vi "InflationApparatus.vi"() -> ()   [LabVIEW 2020]
panel:
  in  "ctrl array":refnum<vi>[](array[refnum])
  in  "camera calibration switch":bool
  in  "force calibration switch":bool
  in  "inflation test switch":bool=TRUE
  in  "dynamic controls":T1(tab)
  in  "stop":bool
  out "current state":string
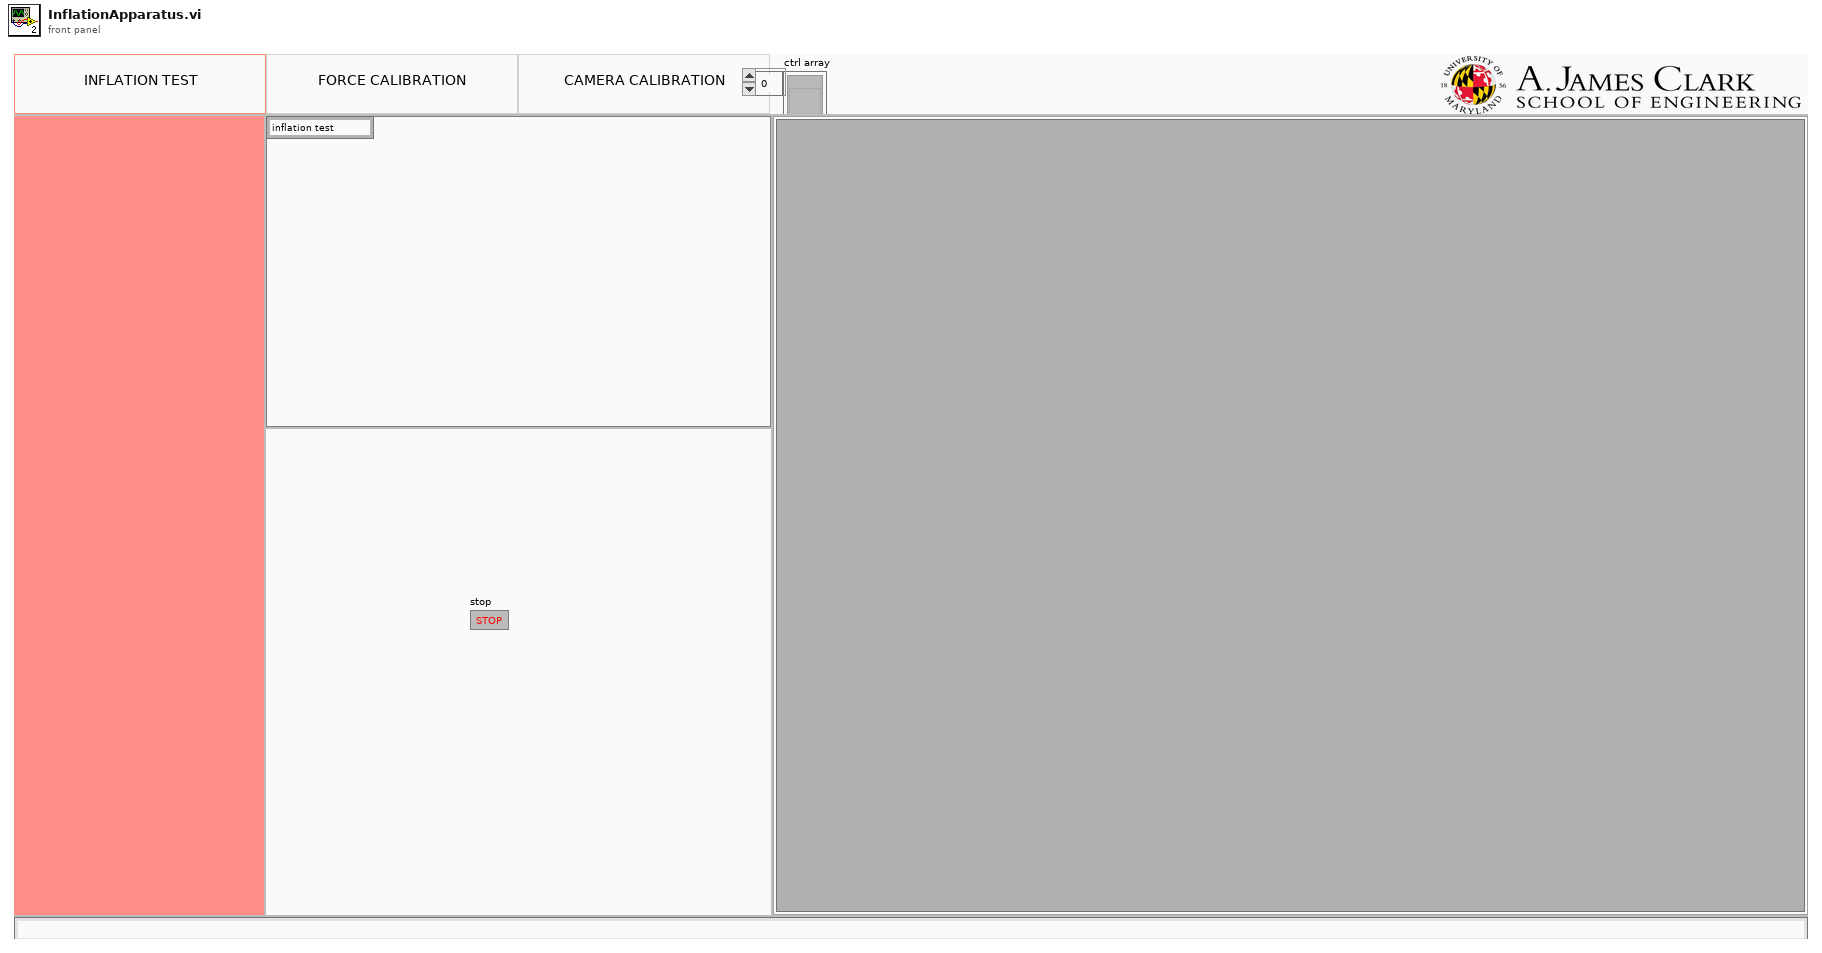
[diagram p1: front panel]
types:
  T1 = enum32{"inflation test", "force calibration", "camera calibration"}
  T2 = enum16{"Share clones between instances", "Preallocate clone for each instance"}
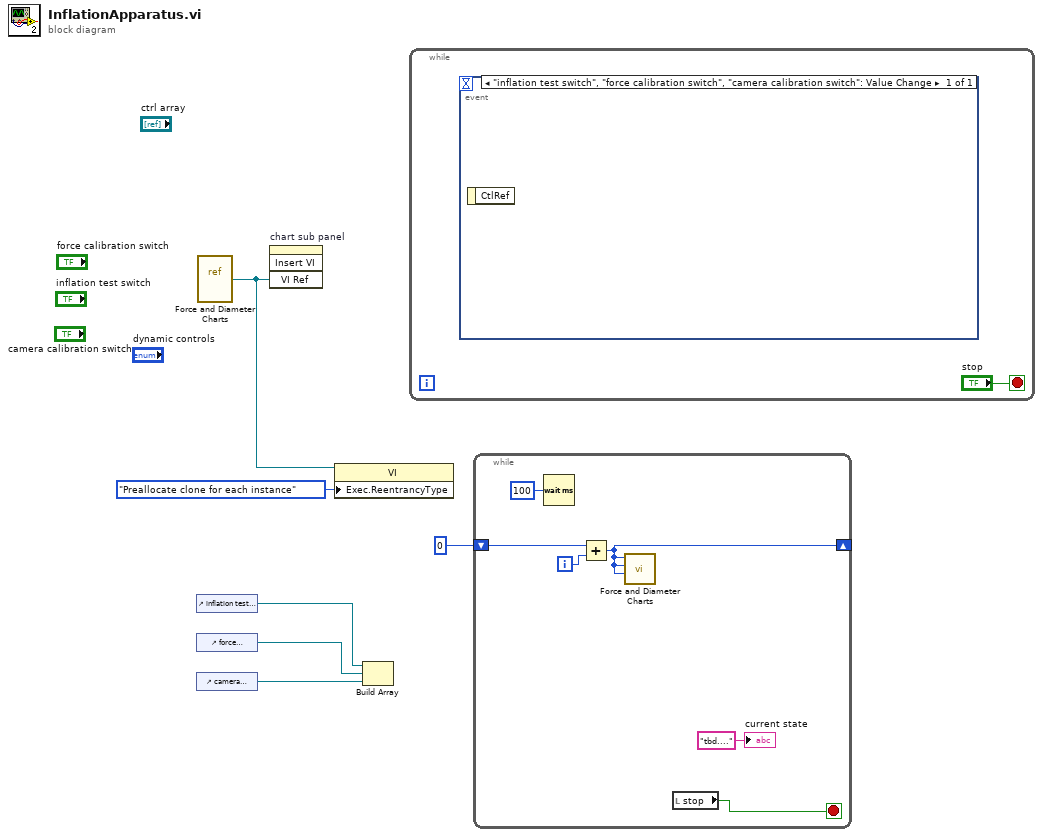
[diagram p0: block diagram]
diagram:
  n1 = control-ref of="inflation test switch"() -> (w3:refnum<vi>)
  n2 = control-ref of="force calibration switch"() -> (w4:refnum<vi>)
  n3 = control-ref of="camera calibration switch"() -> (w5:refnum<vi>)
  n4 = vi-ref "Force and Diameter Charts.vi"() -> (w2:refnum<vi>)
  n5 = invoke on="chart sub panel" class="SubPnl" method="Insert VI"("VI Ref"=w2) -> ()  [unwired: 3 in, 4 out]
  n6 = property class="VI"(reference=w2, "Exec.ReentrancyType"=T2."Preallocate clone for each instance" ("Execution:Reentrancy Type")) -> ()  [unwired: 1 in, 2 out]
  n7 = Build Array(w3, w4, w5) -> ()  [unwired: 1 out]
  n8 = while {
    stop <- "stop" stop-if-true
    n9 = event shown="[0] \"inflation test switch\", \"force calibration switch\", \"camera calibration switch\": Value Change" {
      selector: _ -> [_]
      dyn-events: _ -> [_]
      timeout: _ -> [_]
      event "inflation test switch", "force calibration switch", "camera calibration switch": Value Change {
        n10 = event-data() -> ()  [unwired: 1 in, 1 out]
      }
    }
  }
  n11 = while {
    shift-right: [w10] -> _
    shift-left: 0 -> [w12]
    i -> [w11]
    stop <- w8 stop-if-true
    n12 = Wait (ms)(milliseconds to wait=u32 100) -> ()  [unwired: 1 out]
    n13 = Add(x=w12, y=w11) -> (x+y=w10:i32)
    n14 = call "Force and Diameter Charts.vi"("setpoint"=w10, "force"=w10, "diameter"=w10) -> ()  [unwired: 9 in]
    n15 = local read "stop"() -> (w8:bool)
    "current state" <- "tbd...." ("current state")
  }
